vi "Do.vi"(8 "error in (no error)":errorcluster, 10 "Actor in":refnum<class "Actor.lvclass">, 11 "Go_to_State3 Msg":refnum<class "Go_to_State3 Msg.lvclass">) -> (0 "error out":errorcluster, 2 "Actor out":refnum<class "Actor.lvclass">)   [LabVIEW 2025, in "Demo_States.lvlib" / "Go_to_State3 Msg.lvclass"]
doc: "This VI delivers the message to the actor by calling the appropriate method(s) on the actor."
uses:
  Go_to_State3 Msg.lvclass
  Go_to_State3 Msg.lvclass/Go_to_State3 Msg.ctl
  Demo_States/Demo_States.lvclass
  C:/Program Files (x86)/National Instruments/LabVIEW 2025/vi.lib/ni/Actors/State Actor/State Actor/State Actor.lvclass
  C:/Program Files (x86)/National Instruments/LabVIEW 2025/vi.lib/ActorFramework/Actor/Actor.lvclass
  C:/Users/halstead_rideriver/Documents/Labview_Practice/ATM_Machine_Actor Framework/ATM_ACTORFW/Demo_States/Demo_States/Demo_States.lvclass
  9ef47adc-f318-494c-9b8b-6df3216d6863.vi
  <vilib>/ActorFramework/Actor/Actor.lvclass
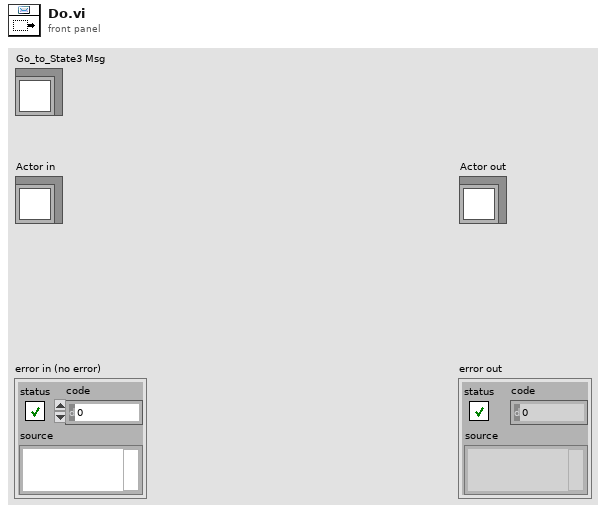
[diagram p1: front panel]
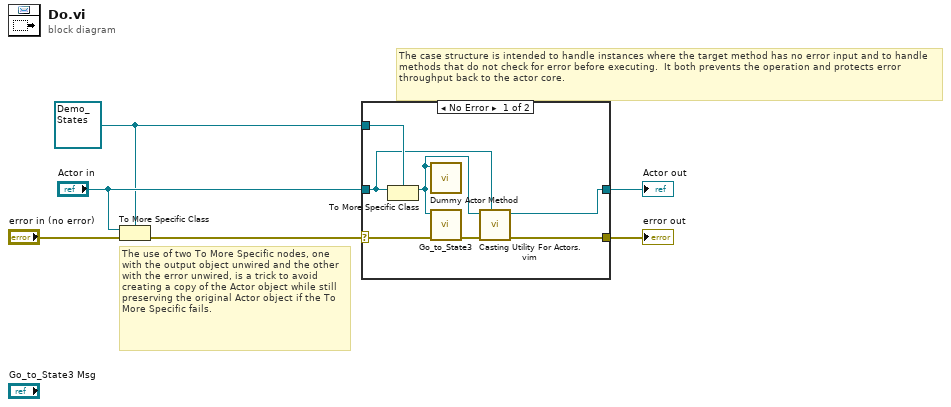
[diagram p0: block diagram]
diagram:
  w1 = refnum<class "Demo_States.lvclass"> refnum ("Actor in")
  # "The use of two To More Specific nodes, one with the output object unwired and the other with the error unwired, is a trick to avoid creating a copy of the Actor object while still preserving the original Actor object if the To More Specific fails."
  # "The case structure is intended to handle instances where the target method has no error input and to handle methods that do not check for error before executing.  It both prevents the operation and protects error throughput back to the actor core."
  n1 = To More Specific Class(target class=w1, reference="Actor in", error in="error in (no error)") -> (error out=w5:errorcluster)  [unwired: 1 out]
  n2 = case shown="No Error" w5 {
    selector: w5 -> [w13 w15]
    tunnel: [w8 w15] -> w4
    tunnel: [w9 w14] -> w3
    tunnel: "Actor in" -> [w10 w14]
    tunnel: w1 -> [w11 _]
    frame No Error {
      n3 = To More Specific Class(target class=w11, reference=w10) -> (specific class reference=w12:refnum<class "Demo_States.lvclass">)  [unwired: 1 in, 1 out]
      n4 = call <resource>:"Dummy Actor Method.vi"("Actor in"=w12) -> ()  [unwired: 9 in, 2 out]
      n5 = call-dynamic "Go_to_State3.vi"("error in (no error)"=w13, "Demo_States in"=w12) -> ("error out"=w7:errorcluster)  [unwired: 8 in, 1 out]
      n6 = call "Casting Utility For Actors.vim"("type"=w10, "error in (no error)"=w7, "Actor in"=w12) -> ("error out"=w8:errorcluster, "Actor out"=w9:refnum<class "Actor.lvclass">)  [unwired: 7 in]
    }
    frame Error {
      # "If type check fails, pass the original object out again."
    }
  }
  "error out" <- w4
  "Actor out" <- w3
